vi "XSubMenu-Init.vi"(3 "Container State":T3, 4 "Previous State":variant, 5 "Previous Version":T2) -> (2 "Current State":T1={"Items"=[{"Tag"="1", "Name"="1", "Symbol"=0, "Checked"=FALSE, "ParentTag"="t"}], "CellHeight"=0})   [LabVIEW 2020, in "XSubMenu.xctl"]
uses:
  XSubMenu.xctl
  XSubMenu-State.ctl
  <vilib>/_xctls/Container State.ctl
  <vilib>/_xctls/Version.ctl
  <vilib>/_xctls/XControlSupport.lvlib
panel:
  in  "Default Indicator State":T1={"Items"=[{"Tag"="1", "Name"="1", "Symbol"=0, "Checked"=FALSE, "ParentTag"="t"}], "CellHeight"=0}
  in  "Default Control State":T1={"Items"=[{"Tag"="1", "Name"="1", "Symbol"=0, "Checked"=FALSE, "ParentTag"="t"}], "CellHeight"=0}
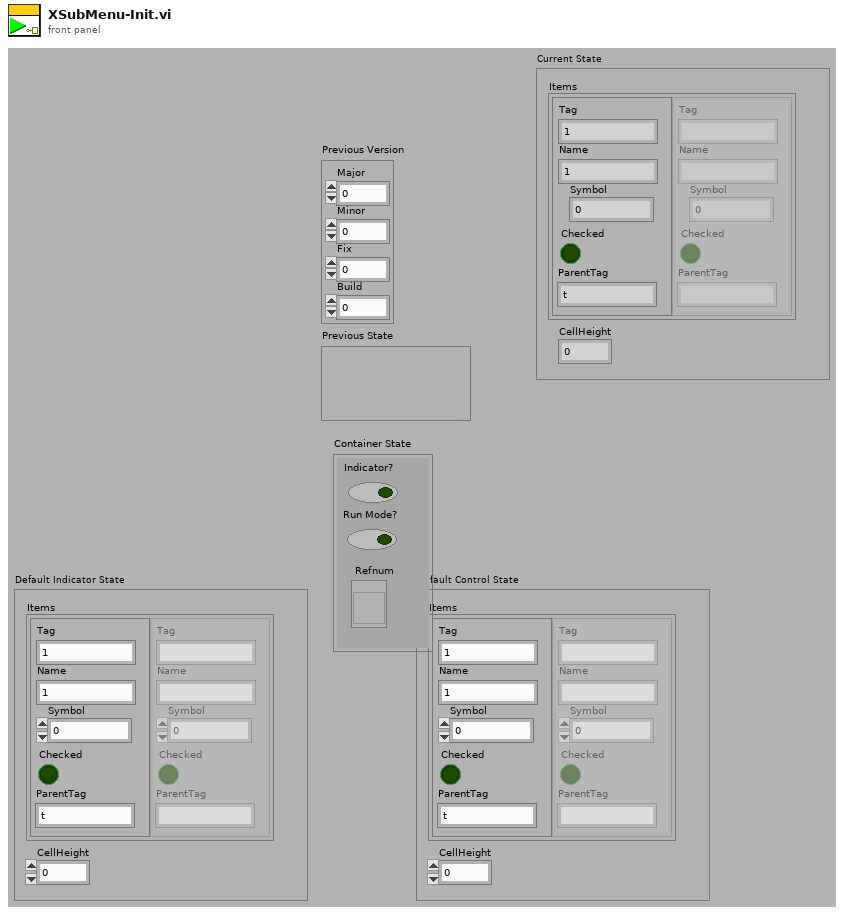
[diagram p1: front panel]
types:
  T1 = typedef "XSubMenu.xctl/XSubMenu-State.ctl" = cluster{"Items":cluster{"Tag":string, "Name":string, "Symbol":i32, "Checked":bool, "ParentTag":string}[], "CellHeight":i32}
  T2 = typedef "XControlSupport.lvlib/Version.ctl" = cluster{"Major":u16, "Minor":u16, "Fix":u16, "Build":u16}
  T3 = typedef "XControlSupport.lvlib/Container State.ctl" = cluster{"Indicator?":bool, "Run Mode?":bool, " Refnum":refnum<vi>}
  T4 = typedef "LVRectTypeDef.ctl" = cluster{"left":i16, "top":i16, "right":i16, "bottom":i16}
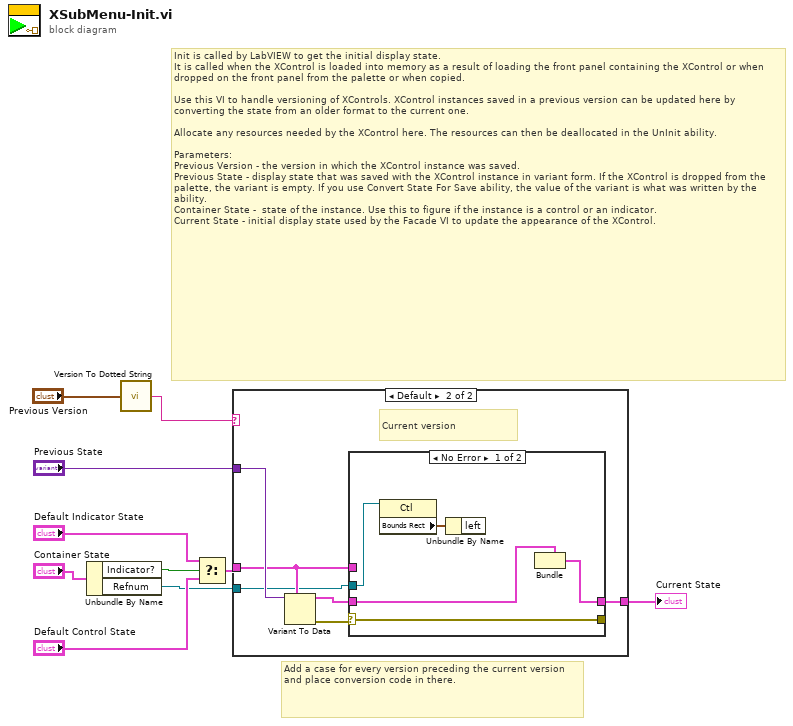
[diagram p0: block diagram]
diagram:
  # "Add a case for every version preceding the current version and place conversion code in there."
  # "Init is called by LabVIEW to get the initial display state.\nIt is called when the XControl is loaded into memory as a result of loading the front panel containing the XControl or when dropped on the front panel from the palette or when copied.\n\nUse this VI to handle versioning of XControls. XControl instances saved in a previous version can be updated here by converting the state from an older format to the current one.\n\nAllocate any resources needed by the XControl here. The resources can then be deallocated in the UnInit ability.\n\nParameters:\nPrevious Version - the version in which the XControl instance was saved.\nPrevious State - display state that was saved with the XControl instance in variant form. If the XControl is dropped from the palette, the variant is empty. If you use Convert State For Save ability, the value of the variant is what was written by the ability. \nContainer State -  state of the instance. Use this to figure if the instance is a control or an indicator.\nCurrent State - initial display state used by the Facade VI to update the appearance of the XControl."
  n1 = Unbundle By Name("Container State") -> ("Indicator?"=w5:bool, "Refnum"=w1:refnum<vi>)
  n2 = call <vilib>:"Version To Dotted String.vi"("Version"="Previous Version") -> ("String Version"=w2:string)
  n3 = Select(t="Default Indicator State", s=w5, f="Default Control State") -> (s? t:f=w4:T1)
  n4 = case shown="Default" w2 {
    tunnel: "Previous State" -> [_ w17]
    tunnel: [w11 w13] -> w9
    tunnel: w4 -> [w11 w14]
    tunnel: w1 -> [_ w12]
    frame "0.0.0.0" {
      # "Just created, use default state"
    }
    frame Default {
      # "Current version"
      n5 = Variant To Data(type=w14, Variant=w17) -> (data=w15:T1, error out=w16:errorcluster)  [unwired: 1 in]
      n6 = case shown="No Error" w16 {
        selector: w16 -> [w22 w23]
        tunnel: w15 -> [w20 _]
        tunnel: [w19 w24] -> w13
        tunnel: w14 -> [_ w24]
        tunnel: [w22 w23] -> _
        tunnel: w12 -> [w21 _]
        frame No Error {
          n7 = property class="Ctl"(reference=w21) -> ("Bounds Rect"=w18:T4)  [unwired: 1 in, 2 out]
          n8 = Unbundle By Name(w18) -> ()  [unwired: 1 out]
          n9 = Bundle(cluster=w20) -> (w19:T1)  [unwired: 2 in]
        }
        frame Error {
          # "Error converting previously \nsaved state. Use default instead."
        }
      }
    }
  }
  "Current State" <- w9
